vi "GFITS_LibGetMemBufPtr.vi"(8 "error in (no error)":errorcluster) -> (0 "error out":errorcluster, 1 "fitssize":i32, 2 "memptr":u64)   [LabVIEW 2016]
uses:
  c/lib/libgfits.so
panel:
  in  "fsize in":i32
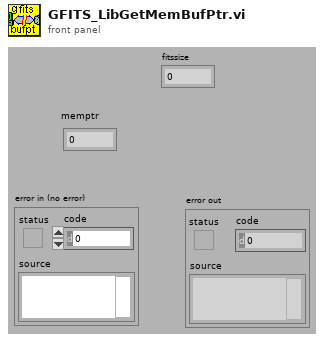
[diagram p1: front panel]
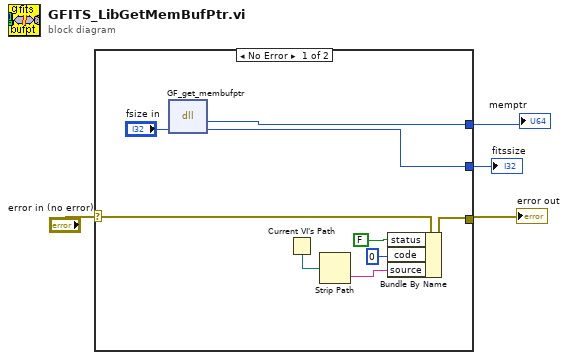
[diagram p0: block diagram]
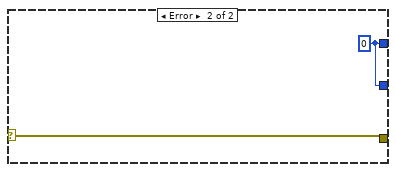
[diagram p2: hidden frame]
diagram:
  n1 = case shown="No Error" "error in (no error)" {
    selector: "error in (no error)" -> [w13 w15]
    tunnel: [w10 w15] -> w3
    tunnel: [w7 w14] -> w2
    tunnel: [w5 w14] -> w1
    frame No Error {
      n2 = dll-call lib="home/simager/panview/PAN/Modules/GFITS/private/c/lib/libgfits.so" fn="GF_get_membufptr"("fitssize"="fsize in") -> ("return type"=w7:u64, "fitssize"=w5:i32)  [unwired: 3 in, 2 out]
      n3 = Current VI's Path() -> (path=w12:path)
      n4 = Strip Path(path=w12) -> (name=w11:string)  [unwired: 1 out]
      n5 = Bundle By Name(cluster=w13, "status"=FALSE, "code"=0, "source"=w11) -> (w10:errorcluster)
    }
    frame Error {
      w14 = u32 0 ("return type")
    }
  }
  "error out" <- w3
  "memptr" <- w2
  "fitssize" <- w1
